vi "DCPower Software-Timed Voltage Sweep.vi"() -> ()   [LabVIEW 2021]
doc: "Demonstrates how to sweep the voltage on a single channel and display the results in a graph. This example performs a software-timed sweep using Single Point source mode. Do not use this example if your device supports Sequence source mode, use the hardware-timed example instead."
uses:
  <instrlib>/niDCPower/nidcpower.llb/niDCPower Source Mode.ctl
  <instrlib>/niDCPower/nidcpower.llb/niDCPower Output Function.ctl
  <instrlib>/niDCPower/nidcpower.llb/niDCPower Wait For Event - Event.ctl
panel:
  in  "Source Delay (Sec)":dbl=0.005
  in  "Points":i32=10 min=1
  in  "Current Limit":dbl=0.01
  out "Current (Amps) vs Voltage (Volts)":cluster{dbl, dbl}[](graph)
  in  "Voltage Level Stop":dbl=5.0
  in  "Voltage Level Start":dbl=1.0
  in  "Channel Name":string="0"
  in  "Resource Name":refnum<k15>="DCPOWER0" caption="Resource Name*"
  # "Overview: This example demonstrates how to sweep the voltage on a single channel and display the results in a graph.  \nThis example performs a software-timed sweep using Single Point source mode.  If your device supports Sequence Source \nmode, it is recommended that you use the hardware-timed example instead.\nRequirements: NI-DCPower\nInstructions:\n1. Select the appropriate device in the Resource Name control.\n2. Configure the parameters of the sweep.\n3. Run the VI."
  # "*must manutally enter, DCPower device will not be found\nin drop down"
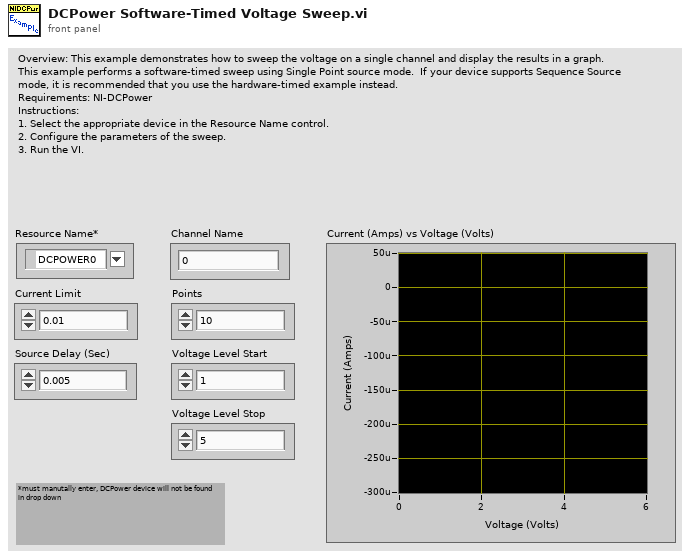
[diagram p1: front panel]
types:
  T1 = typedef "niDCPower Output Function.ctl" = i32
  T2 = typedef "niDCPower Source Mode.ctl" = i32
  T3 = typedef "niDCPower Wait For Event - Event.ctl" = i32
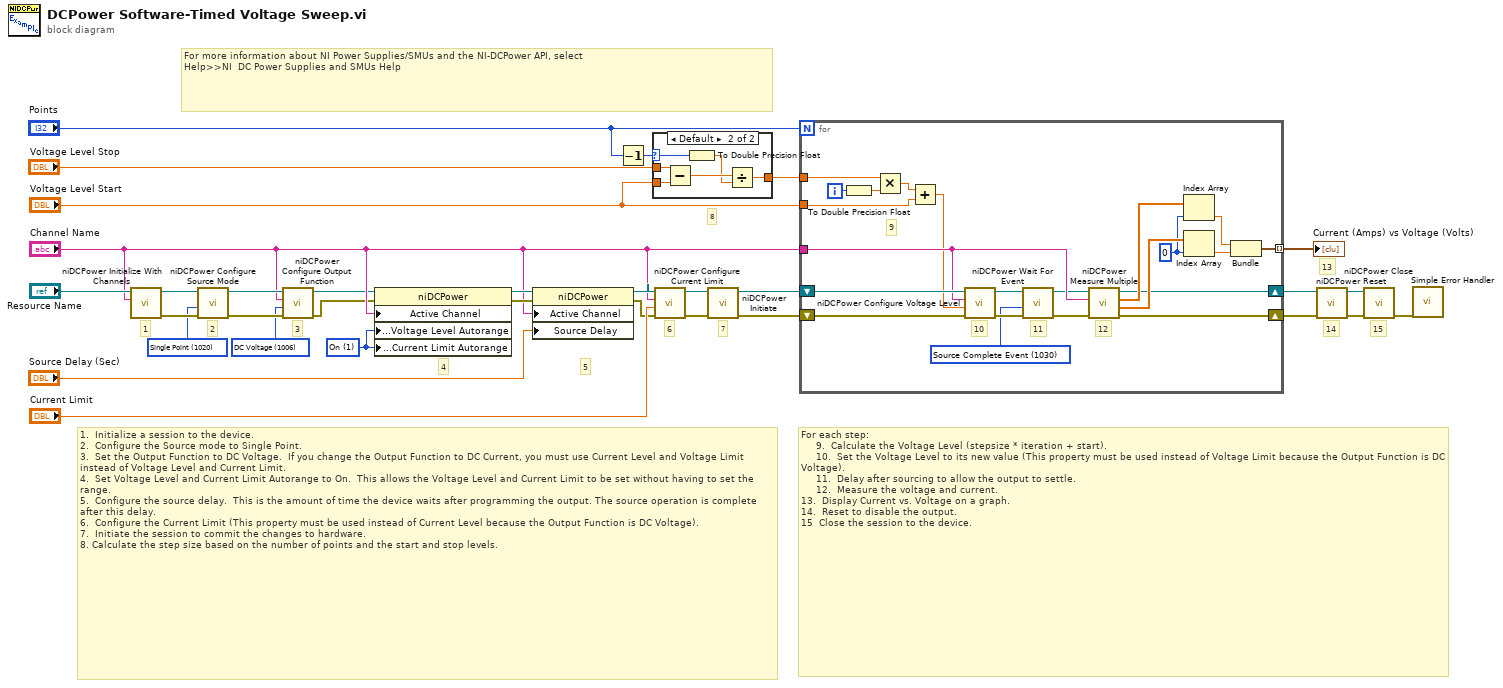
[diagram p0: block diagram]
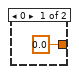
[diagram p2: hidden frame]
diagram:
  w1 = T1 1006 items=["DC Voltage"=1006, "DC Current"=1007, "Pulse Voltage"=1049, "Pulse Current"=1050] ("output function")
  w11 = T2 1020 items=["Single Point"=1020, "Sequence"=1021] ("source mode")
  w2 = 1 items=["Off", "On"] ("DC Voltage:Voltage Level Autorange")
  # "For more information about NI Power Supplies/SMUs and the NI-DCPower API, select\nHelp>>NI  DC Power Supplies and SMUs Help"
  # "5"
  # "8"
  # "3"
  # "1.  Initialize a session to the device.\n2.  Configure the Source mode to Single Point.\n3.  Set the Output Function to DC Voltage.  If you change the Output Function to DC Current, you must use Current Level and Voltage Limit instead of Voltage Level and Current Limit.\n4.  Set Voltage Level and Current Limit Autorange to On.  This allows the Voltage Level and Current Limit to be set without having to set the range.\n5.  Configure the source delay.  This is the amount of time the device waits after programming the output. The source operation is complete after this delay.\n6.  Configure the Current Limit (This property must be used instead of Current Level because the Output Function is DC Voltage).\n7.  Initiate the session to commit the changes to hardware.\n8. Calculate the step size based on the number of points and the start and stop levels."
  # "4"
  # "6"
  # "13"
  # "15"
  # "14"
  # "7"
  # "2"
  # "1"
  # "For each step:\n     9.  Calculate the Voltage Level (stepsize * iteration + start).    \n     10.  Set the Voltage Level to its new value (This property must be used instead of Voltage Limit because the Output Function is DC Voltage). \n     11.  Delay after sourcing to allow the output to settle.\n     12.  Measure the voltage and current. \n13.  Display Current vs. Voltage on a graph.\n14.  Reset to disable the output.\n15  Close the session to the device."
  n1 = call <instrlib>:"niDCPower Initialize With Channels.vi"("channels"="Channel Name", "resource name"="Resource Name") -> ("error out"=w15:errorcluster, "instrument handle out"=w13:refnum<k15>)  [unwired: 3 in, 5 out]
  n2 = call <instrlib>:"niDCPower Configure Source Mode.vi"("error in (no error)"=w15, "source mode"=w11, "instrument handle"=w13) -> ("error out"=w14:errorcluster, "instrument handle out"=w12:refnum<k15>)  [unwired: 7 out]
  n3 = call <instrlib>:"niDCPower Configure Output Function.vi"("error in (no error)"=w14, "output function"=w1, "channel name"="Channel Name", "instrument handle"=w12) -> ("error out"=w3:errorcluster, "instrument handle out"=w4:refnum<k15>)  [unwired: 6 out]
  n4 = property class="niDCPower"(reference=w4, error in=w3, "Active Channel"="Channel Name", "Source:DC Voltage:Voltage Level Autorange"=w2, "Source:DC Voltage:Current Limit Autorange"=w2) -> (reference out=w10:refnum<k15>, error out=w7:errorcluster)
  n5 = property class="niDCPower"(reference=w10, error in=w7, "Active Channel"="Channel Name", "Source Delay"="Source Delay (Sec)") -> (reference out=w9:refnum<k15>, error out=w8:errorcluster)
  n6 = Decrement(x="Points") -> (x-1=w19:i32)
  n7 = case shown="Default" w19 {
    selector: w19 -> [_ w35]
    tunnel: "Voltage Level Stop" -> [_ w38]
    tunnel: [0.0 w37] -> w21
    tunnel: "Voltage Level Start" -> [_ w36]
    frame 0 {
    }
    frame Default {
      n8 = Subtract(x=w38, y=w36) -> (x-y=w39:dbl)
      n9 = To Double Precision Float(number=w35) -> (double precision float=w34:dbl)
      n10 = Divide(x=w39, y=w34) -> (x/y=w37:dbl)
    }
  }
  n11 = call <instrlib>:"niDCPower Configure Current Limit.vi"("error in (no error)"=w8, "current limit"="Current Limit", "channel name"="Channel Name", "instrument handle"=w9) -> ("error out"=w17:errorcluster, "instrument handle out"=w16:refnum<k15>)  [unwired: 6 out]
  n12 = call <instrlib>:"niDCPower Initiate.vi"("error in (no error)"=w17, "instrument handle"=w16) -> ("error out"=w26:errorcluster, "instrument handle out"=w27:refnum<k15>)  [unwired: 8 out]
  n13 = for {
    N: "Points" -> [_]
    tunnel: [w59] -> w22 mode=indexing
    shift-right: [w57] -> w23
    shift-left: w26 -> [w60]
    tunnel: w21 -> [w51]
    tunnel: "Voltage Level Start" -> [w47]
    shift-right: [w52] -> w24
    shift-left: w27 -> [w61]
    tunnel: "Channel Name" -> [w58]
    i -> [w50]
    w41 = T3 1030 items=["Source Complete Event"=1030, "Measure Complete Event"=1031, "Sequence Iteration Complete Event"=1032, "Sequence Engine Done Event"=1033] ("event")
    w40 = 0 ("index")
    # "11"
    # "12"
    # "10"
    # "9"
    n14 = To Double Precision Float(number=w50) -> (double precision float=w49:dbl)
    n15 = Multiply(x=w51, y=w49) -> (x*y=w48:dbl)
    n16 = Add(x=w48, y=w47) -> (x+y=w46:dbl)
    n17 = call <instrlib>:"niDCPower Configure Voltage Level.vi"("error in (no error)"=w60, "voltage level"=w46, "channel name"=w58, "instrument handle"=w61) -> ("error out"=w45:errorcluster, "instrument handle out"=w42:refnum<k15>)  [unwired: 6 out]
    n18 = call <instrlib>:"niDCPower Wait For Event.vi"("error in (no error)"=w45, "event"=w41, "instrument handle"=w42) -> ("error out"=w44:errorcluster, "instrument handle out"=w43:refnum<k15>)  [unwired: 1 in, 6 out]
    n19 = call <instrlib>:"niDCPower Measure Multiple.vi"("error in (no error)"=w44, "channel name"=w58, "instrument handle"=w43) -> ("error out"=w57:errorcluster, "current measurements"=w56:dbl[], "voltage measurements"=w55:dbl[], "instrument handle out"=w52:refnum<k15>)  [unwired: 5 out]
    n20 = Index Array(array=w55, index=w40) -> (element=w54:dbl)
    n21 = Index Array(array=w56, index=w40) -> (element=w53:dbl)
    n22 = Bundle(w54, w53) -> (w59:cluster{dbl, dbl})  [unwired: 1 out]
  }
  "Current (Amps) vs Voltage (Volts)" <- w22
  n23 = call <instrlib>:"niDCPower Reset.vi"("error in (no error)"=w23, "instrument handle"=w24) -> ("error out"=w31:errorcluster, "instrument handle out"=w30:refnum<k15>)  [unwired: 8 out]
  n24 = call <instrlib>:"niDCPower Close.vi"("error in (no error)"=w31, "instrument handle"=w30) -> ("error out"=w29:errorcluster)  [unwired: 9 out]
  n25 = call <vilib>:"Simple Error Handler.vi"("error in (no error)"=w29) -> ()  [unwired: 1 in, 8 out]
